vi "Handshake_PreUUT.vi"(8 "error in":errorcluster, 9 "Tester Tx":T2={"Fault"=FALSE, "StepNo"=0, "Ready"=TRUE, "HighVoltage"=FALSE, "TestRunning"=FALSE, "ResultsReady"=FALSE, "Results"=0, "ElapsedTime"=0, "Online"=TRUE, "TimeCompleted"=[], "Timeout"=FALSE, "Heartbeat"=FALSE}, 10 "Tester Rx In":T1={"Start"=FALSE, "NestStatus"=FALSE, "PalletID"=0, "BarcodeData"="P:10-000001R:04S:QMC2200001", "StepEcho"=0, "Cylinder_1"=FALSE, "Cylinder_2"=FALSE, "Cylinder_3"=FALSE, "Cylinder_4"=FALSE, "Cylinder_5"=FALSE, "ResultsAck"=FALSE, "Reset"=FALSE, "Stop"=FALSE, "FaultCode"=0}) -> (0 "error out":errorcluster, 2 "Tester Rx out":T1)   [LabVIEW 2019, in "Station Actor.lvlib" / "Station Actor.lvclass"]
uses:
  Station Actor.lvclass
  Custom Controls/Tester Rx Dataset.ctl
  Custom Controls/Tester Tx Dataset.ctl
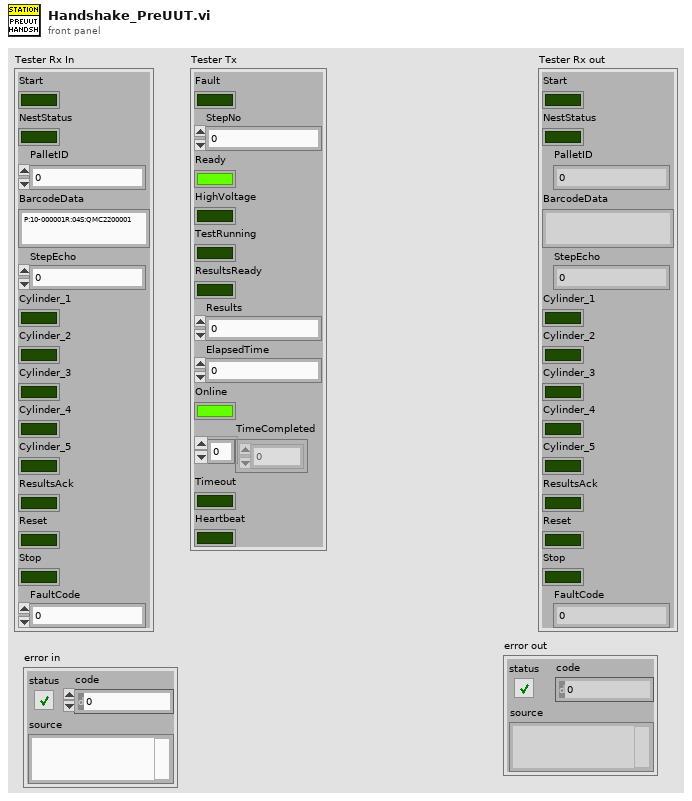
[diagram p1: front panel]
types:
  T1 = typedef "Station Actor.lvlib/Station Actor.lvclass/Tester Rx Dataset.ctl" = cluster{"Start":bool, "NestStatus":bool, "PalletID":u32, "BarcodeData":string, "StepEcho":u32, "Cylinder_1":bool, "Cylinder_2":bool, "Cylinder_3":bool, "Cylinder_4":bool, "Cylinder_5":bool, "ResultsAck":bool, "Reset":bool, "Stop":bool, "FaultCode":u32}
  T2 = typedef "Station Actor.lvlib/Station Actor.lvclass/Tester Tx Dataset.ctl" = cluster{"Fault":bool, "StepNo":u32, "Ready":bool, "HighVoltage":bool, "TestRunning":bool, "ResultsReady":bool, "Results":u32, "ElapsedTime":u32, "Online":bool, "TimeCompleted":i32[], "Timeout":bool, "Heartbeat":bool}
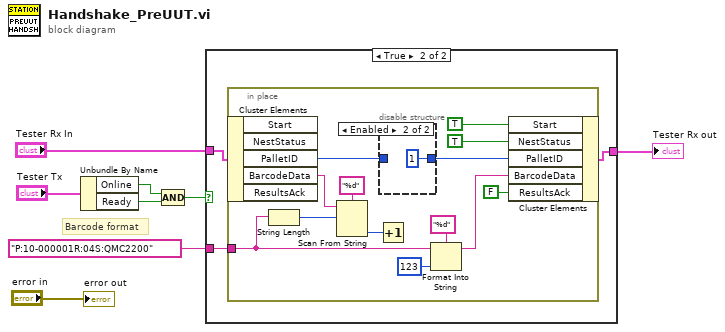
[diagram p0: block diagram]
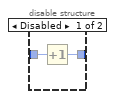
[diagram p3: hidden frame]
diagram:
  # "Barcode format"
  n1 = Unbundle By Name("Tester Tx") -> ("Online"=w2:bool, "Ready"=w3:bool)
  n2 = Compound Arithmetic op=AND(w2, w3) -> (w1:bool)
  n3 = case shown="True" w1 {
    tunnel: "Tester Rx In" -> [w9 w12]
    tunnel: [w9 w11] -> w5
    tunnel: "P:10-000001R:04S:QMC2200" -> [_ w10]
    frame False {
    }
    frame True {
      n4 = in-place {
        in-place-border: w10 -> [w16]
        n5 = in-place-cluster #1(w12) -> ("PalletID"=w23:u32, "BarcodeData"=w15:string)  [unwired: 3 out]
        n6 = String Length(string=w16) -> (length=w19:i32)
        n7 = Scan From String(format string="%d", input string=w15, initial scan location=w19) -> (output 1=w18:i32)  [unwired: 2 in, 3 out]
        n8 = Increment(x=w18) -> ()  [unwired: 1 out]
        n9 = disable-structure shown="Enabled" {
          disable-tunnel: w23 -> [w27 _]
          disable-tunnel: [w26 u32 1] -> w22
          frame Disabled {
            n10 = Increment(x=w27) -> (x+1=w26:u32)
          }
          frame Enabled {
          }
        }
        n11 = Format Into String(format string="%d", initial string=w16, 123 ("input 1")) -> (resulting string=w17:string)  [unwired: 1 in, 1 out]
        n12 = in-place-cluster #1("Start"=TRUE, "NestStatus"=TRUE, "PalletID"=w22, "BarcodeData"=w17, "ResultsAck"=FALSE) -> (w11:T1)
      }
    }
  }
  "Tester Rx out" <- w5
  "error out" <- "error in"
